vi "Read FXP.vi"(7 "FXP Configuration":T1, 8 "error in":errorcluster, 10 "register name":string, 11 "session in":u32) -> (0 "error out":errorcluster, 2 "DBL Value":dbl, 3 "session out":u32)   [LabVIEW 2018, in "Scalar IO Operations.lvlib"]
uses:
  Scalar IO Operations.lvlib
  TypeDefs/FXP Configuration.ctl
  <vilib>/fxp/LVFixedPointRepBitsTypeDef.ctl
  <vilib>/fxp/LVFixedPointRepRangeTypeDef.ctl
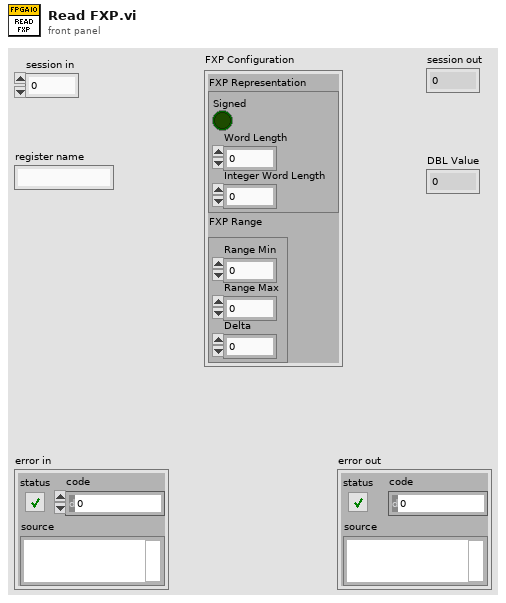
[diagram p1: front panel]
types:
  T1 = typedef "Scalar IO Operations.lvlib/FXP Configuration.ctl" = cluster{"FXP Representation":T2, "FXP Range":T3}
  T2 = typedef "LVFixedPointRepBitsTypeDef.ctl" = cluster{"Signed":bool, "Word Length":u32, "Integer Word Length":i32}
  T3 = typedef "LVFixedPointRepRangeTypeDef.ctl" = cluster{"Range Min":dbl, "Range Max":dbl, "Delta":dbl}
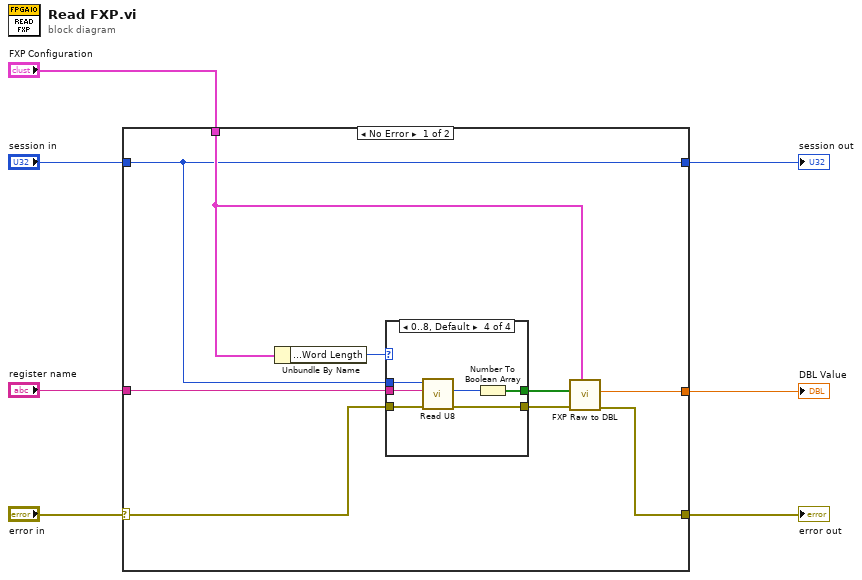
[diagram p0: block diagram]
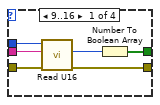
[diagram p2: hidden frame]
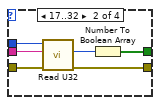
[diagram p3: hidden frame]
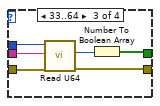
[diagram p4: hidden frame]
diagram:
  n1 = case shown="No Error" "error in" {
    selector: "error in" -> [w9 w42]
    tunnel: "session in" -> [w11 w41]
    tunnel: [w16 w42] -> w7
    tunnel: "register name" -> [w14 _]
    tunnel: [w11 w41] -> w6
    tunnel: [w15 _] -> w5
    tunnel: "FXP Configuration" -> [w12 _]
    frame No Error {
      n2 = Unbundle By Name(w12) -> ("FXP Representation.Word Length"=w13:u32)
      n3 = case shown="0..8, Default" w13 {
        tunnel: w14 -> [w20 w26 w32 w39]
        tunnel: [w17 w23 w30 w40] -> w8
        tunnel: w11 -> [w21 w27 w33 w38]
        tunnel: [w19 w25 w29 w36] -> w10
        tunnel: w9 -> [w22 w28 w34 w35]
        frame 9..16 {
          n4 = call "Read U16.vi"("error in"=w22, "register name"=w20, "session in"=w21) -> ("error out"=w19:errorcluster, "value out"=w18:u16)  [unwired: 6 in, 1 out]
          n5 = Number To Boolean Array(number=w18) -> (Boolean array=w17:bool[])
        }
        frame 17..32 {
          n6 = call "Read U32.vi"("error in"=w28, "register name"=w26, "session in"=w27) -> ("error out"=w25:errorcluster, "value out"=w24:u32)  [unwired: 6 in, 1 out]
          n7 = Number To Boolean Array(number=w24) -> (Boolean array=w23:bool[])
        }
        frame 33..64 {
          n8 = call "Read U64.vi"("error in"=w34, "register name"=w32, "session in"=w33) -> ("error out"=w29:errorcluster, "value out"=w31:u64)  [unwired: 6 in, 1 out]
          n9 = Number To Boolean Array(number=w31) -> (Boolean array=w30:bool[])
        }
        frame 0..8, Default {
          n10 = call "Read U8.vi"("error in"=w35, "register name"=w39, "session in"=w38) -> ("error out"=w36:errorcluster, "value out"=w37:u8)  [unwired: 6 in, 1 out]
          n11 = Number To Boolean Array(number=w37) -> (Boolean array=w40:bool[])
        }
      }
      n12 = call "FXP Raw to DBL.vi"("FXP Configuration"=w12, "error in (no error)"=w10, "Bool Data"=w8) -> ("error out"=w16:errorcluster, "DBL Value"=w15:dbl)  [unwired: 7 in]
    }
    frame Error {
    }
  }
  "error out" <- w7
  "session out" <- w6
  "DBL Value" <- w5
